vi "solar_voy Register (Hide).vi"(5 "CMD":enum8{"CMD", "TLM"}(ring), 6 "Suppress Errors? (T)":bool=TRUE, 7 "TARGET":string, 8 "error in (no error)":errorcluster, 9 "Hide? (F)":bool, 10 "PACKET":string, 11 "Voyager Refnum in":T1) -> (0 "error out":errorcluster, 3 "Voyager Refnum out":T1)   [LabVIEW 2018]
doc: "This hides a Voyager packet during export. This is usefull for registering internal commands that should not be commandable from COSMOS."
uses:
  solar_voy_ctl Voyager Refnum.ctl
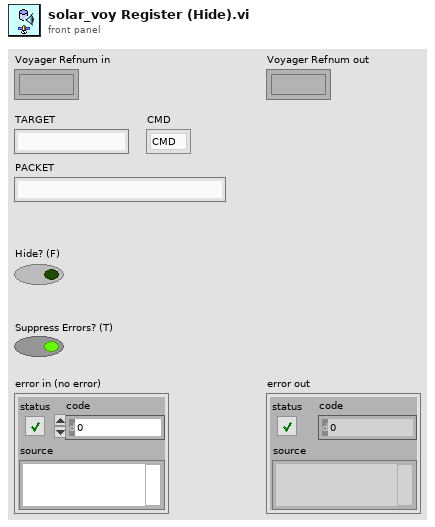
[diagram p1: front panel]
types:
  T1 = typedef "solar_voy_ctl Voyager Refnum.ctl" = refnum<k1>
  T2 = typedef "solar_voy_ctl Voyager.ctl" = cluster{"PACKETS":T3[], "COSMOS_Root":path, "CMD_HDR":T8, "TLM_HDR":T8, "TCPs":T9[], "VoyagerIDOffset":cluster{"VoyagerIDOffset":u16[], "Target Names":string[]}}
  T3 = typedef "solar_voy_def_ctl PACKET.ctl" = cluster{"PACKET_ID":T4, "ENDIAN":enum8{"BIG", "LITTLE"}, "DESC":string, "HZRD":bool, "ITEMS":T5[], "NoExport":bool, "last_time":timestamp, "last_count":u32, "last_data":string}
  T4 = typedef "solar_voy_def_ctl PACKET_ID.ctl" = cluster{"ID":u16, "CMD":enum8{"CMD", "TLM"}, "TARGET":string, "PACKET":string}
  T5 = typedef "solar_voy_def_ctl ITEM.ctl" = cluster{"NAME":string, "OFFSET":i32, "SIZE":i32, "TYPE":T6, "EACH_SIZE":i32, "LVTYPE":T7, "MIN":dbl, "MAX":dbl, "DEFAULT":string, "DESC":string, "ID":bool, "MODIFIERS":variant, "last_value":variant}
  T6 = typedef "solar_voy_def_ctl ITEM TYPE.ctl" = enum8{"BLOCK", "INT", "UINT", "FLOAT", "STRING"}
  T7 = typedef "solar_type Item Type.ctl" = enum16{"NULL", "UNKNOWN", "CLUSTER", "I8", "I16", "I32", "I64", "U8", "U16", "U32", "U64", "U8_ENUM", "U16_ENUM", "U32_ENUM", "SGL", "DBL", "BOOLEAN", "STRING", "PATH", "VISA", "TAG", "TIME", "I8_1D", "I16_1D", "I32_1D", "I64_1D", "U8_1D", "U16_1D", "U32_1D", "U64_1D", "U8_ENUM_1D", "U16_ENUM_1D", "U32_ENUM_1D", "SGL_1D", "DBL_1D", "BOOLEAN_1D", "STRING_1D", "PATH_1D", "VISA_1D", "TAG_1D", "TIME_1D", "I8_2D", "I16_2D", "I32_2D", "I64_2D", "U8_2D", "U16_2D", "U32_2D", "U64_2D", "U8_ENUM_2D", "U16_ENUM_2D", "U32_ENUM_2D", "SGL_2D", "DBL_2D", "BOOLEAN_2D", "STRING_2D", "PATH_2D", "VISA_2D", "TAG_2D", "TIME_2D"}
  T8 = typedef "solar_voy_def_ctl HDR.ctl" = cluster{"ITEMS":T5[], "LENGTH_NAME":string, "LENGTH_VALUE_OFFSET":i32, "ID_NAME":string, "ENDIAN":enum8{"BIG", "LITTLE"}, "GUID_NAME":string, "DEFAULT_TARGET":string, "DEFAULT_PACKET":string, "DEFAULT_ERROR":string}
  T9 = typedef "solar_voy_ctl TCP.ctl" = cluster{"Connected":bool, "Port":u16, "Listener":refnum<k5>, "ServerIP":string, "TCP":refnum<k5>, "Setup":T10, "VIRefnum":refnum<vi>, "TARGETS_CMD":string[], "TARGETS_TLM":string[]}
  T10 = typedef "solar_voy_ctl Port Setup.ctl" = enum8{"SERVER", "CLIENT", "SERVER_CMD", "SERVER_TLM"}
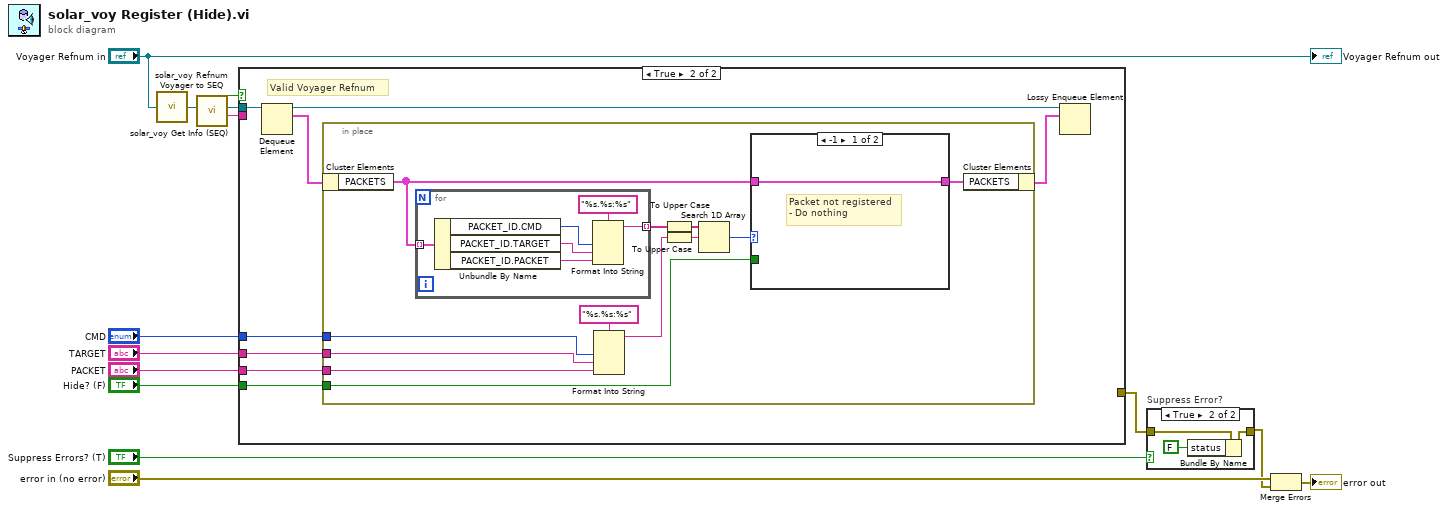
[diagram p0: block diagram]
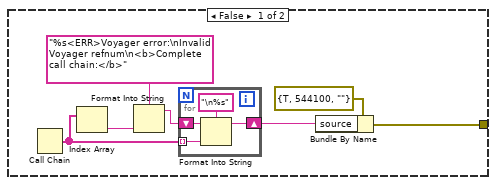
[diagram p2: hidden frame]
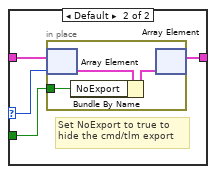
[diagram p3: hidden frame]
diagram:
  n1 = call "solar_voy Refnum Voyager to SEQ.vi"("Voyager Refnum"="Voyager Refnum in") -> ("Voyager SEQ"=w14:refnum<queue>)
  n2 = call "solar_voy Get Info (SEQ).vi"("Voyager SEQ in"=w14) -> ("Interface Name"=w12:string, "Voyager SEQ out"=w13:refnum<queue>, "Valid?"=w11:bool)  [unwired: 8 in]
  n3 = case shown="True" w11 {
    tunnel: w13 -> [_ w32]
    tunnel: w12 -> [_ _]
    tunnel: [w15 _] -> w8
    tunnel: "Hide? (F)" -> [_ w29]
    tunnel: "CMD" -> [_ w28]
    tunnel: "TARGET" -> [_ w27]
    tunnel: "PACKET" -> [_ w26]
    frame False {
      n4 = Call Chain() -> (call chain=w18:string[])
      n5 = Index Array(array=w18) -> (element=w20:string)  [unwired: 1 in]
      n6 = Format Into String(format string="%s<ERR>Voyager error:\nInvalid Voyager refnum\n<b>Complete call chain:</b>", w20) -> (resulting string=w19:string)  [unwired: 2 in, 1 out]
      n7 = for {
        tunnel: w18 -> [w25] mode=indexing
        shift-right: [w24] -> w17
        shift-left: w19 -> [w23]
        n8 = Format Into String(format string="\n%s", initial string=w23, w25) -> (resulting string=w24:string)  [unwired: 1 in, 1 out]
      }
      n9 = Bundle By Name(cluster=errorcluster {"status"=TRUE, "code"=544100, "source"=""} ("error in (no error)"), "source"=w17) -> (w15:errorcluster)
    }
    frame True {
      # "Valid Voyager Refnum"
      n10 = Dequeue Element(queue=w32) -> (queue out=w33:refnum<queue>, element=w31:T2)  [unwired: 2 in, 2 out]
      n11 = in-place {
        in-place-border: w29 -> [w37]
        in-place-border: w28 -> [w36]
        in-place-border: w27 -> [w35]
        in-place-border: w26 -> [w34]
        n12 = in-place-cluster #1(w31) -> ("PACKETS"=w38:T3[])
        n13 = for {
          tunnel: w38 -> [w55] mode=indexing
          tunnel: [w54] -> w45 mode=indexing
          n14 = Unbundle By Name(w55) -> ("PACKET_ID.CMD"=w57:enum8{"CMD", "TLM"}, "PACKET_ID.TARGET"=w58:string, "PACKET_ID.PACKET"=w59:string)
          n15 = Format Into String(format string="%s.%s:%s", w57, w58, w59) -> (resulting string=w54:string)  [unwired: 2 in, 1 out]
        }
        n16 = Format Into String(format string="%s.%s:%s", w36, w35, w34) -> (resulting string=w43:string)  [unwired: 2 in, 1 out]
        n17 = To Upper Case(1:w45) -> (0:w41:string[])
        n18 = To Upper Case(1:w43) -> (0:w44:string)
        n19 = Search 1D Array(1D array=w41, element=w44) -> (index of element=w40:i32)  [unwired: 1 in]
        n20 = case shown="-1" w40 {
          selector: w40 -> [_ w49]
          tunnel: [w46 w48] -> w39
          tunnel: w38 -> [w46 w50]
          tunnel: w37 -> [_ w47]
          frame -1 {
            # "Packet not registered\n- Do nothing"
          }
          frame Default {
            # "Set NoExport to true to\nhide the cmd/tlm export"
            n21 = in-place {
              in-place-border: w47 -> [w51]
              n22 = in-place-array #2(w50, w49) -> (w53:T3)
              n23 = Bundle By Name(cluster=w53, "NoExport"=w51) -> (w52:T3)
              n24 = in-place-array #2(w52) -> (w48:T3[])  [unwired: 1 out]
            }
          }
        }
        n25 = in-place-cluster #1("PACKETS"=w39) -> (w30:T2)
      }
      n26 = Lossy Enqueue Element(queue=w33, element=w30) -> ()  [unwired: 1 in, 4 out]
    }
  }
  n27 = case "Suppress Error?" shown="True" "Suppress Errors? (T)" {
    tunnel: w8 -> [w60 w63]
    tunnel: [w60 w62] -> w6
    frame False {
    }
    frame True {
      n28 = Bundle By Name(cluster=w63, "status"=FALSE) -> (w62:errorcluster)
    }
  }
  n29 = Merge Errors("error in (no error)", w6) -> (→"error out":errorcluster)
  "Voyager Refnum out" <- "Voyager Refnum in"
